vi "read_timer_holding_time.vi"(8 "error in (no error)":errorcluster, 11 "config_file_name":string) -> (0 "error out":errorcluster, 2 "values":cluster{"holding time":dbl}, 3 "config_file_name_out":string)   [LabVIEW 2015]
uses:
  <vilib>/Utility/config.llb/Read Key (String).vi
  <vilib>/Utility/config.llb/NI_LVConfig.lvlib
panel:
  # "Devuelve datos de la sección TIMER del archivo de configuración"
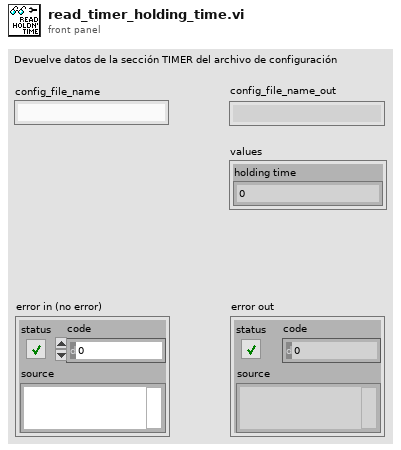
[diagram p1: front panel]
types:
  T1 = typedef "NI_LVConfig.lvlib/Config Data RefNum.ctl" = refnum<k1>
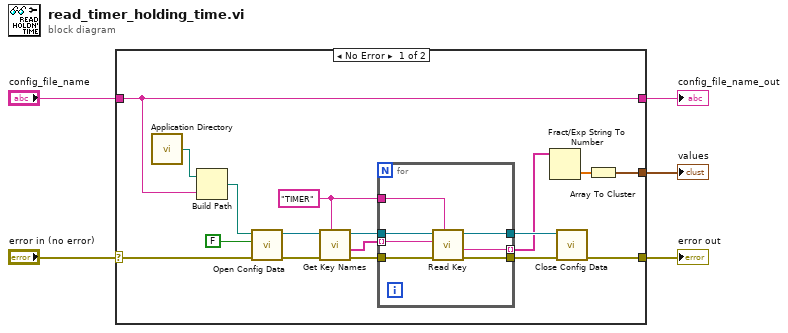
[diagram p0: block diagram]
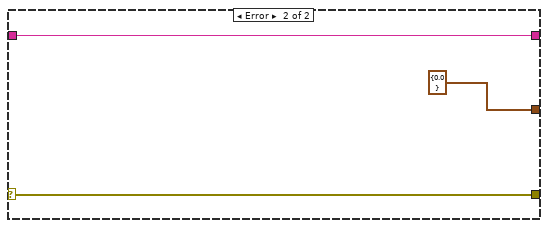
[diagram p2: hidden frame]
diagram:
  n1 = case shown="No Error" "error in (no error)" {
    selector: "error in (no error)" -> [w13 w32]
    tunnel: [w12 w32] -> w5
    tunnel: [w11 w31] -> w3
    tunnel: "config_file_name" -> [w11 w31]
    tunnel: [w6 cluster{"[0]":dbl} {"[0]"=0.0}] -> w1
    frame No Error {
      w18 = "TIMER" ("section")
      n2 = call <vilib>:"Application Directory.vi"() -> ("Application Directory"=w20:path)
      n3 = Build Path(base path=w20, name or relative path=w11) -> (appended path=w19:path)
      n4 = call <vilib>:"Open Config Data.vi"("error in (no error)"=w13, "create file if necessary (T)"=FALSE, "configuration file path"=w19) -> ("error out"=w22:errorcluster, "refnum"=w21:T1)  [unwired: 6 in, 1 out]
      n5 = call <vilib>:"Get Key Names.vi"("section"=w18, "error in (no error)"=w22, "refnum"=w21) -> ("error out"=w16:errorcluster, "key names"=w10:string[], "refnum out"=w17:T1)  [unwired: 5 in, 1 out]
      n6 = for {
        tunnel: w10 -> [w29] mode=indexing
        tunnel: [w28] -> w8 mode=indexing
        tunnel: w18 -> [w27]
        tunnel: w17 -> [w26]
        tunnel: w16 -> [w25]
        tunnel: [w24] -> w15
        tunnel: [w23] -> w14
        n7 = call-poly <vilib>:"Read Key.vi"("section"=w27, "error in (no error)"=w25, "key"=w29, "refnum"=w26) -> ("error out"=w23:errorcluster, "value"=w28:string, "refnum out"=w24:T1)  [unwired: 4 in, 1 out]
      }
      n8 = Fract/Exp String To Number(string=w8) -> (number=w7:dbl[])  [unwired: 3 in, 1 out]
      n9 = call <vilib>:"Close Config Data.vi"("error in (no error)"=w14, "refnum"=w15) -> ("error out"=w12:errorcluster)  [unwired: 8 in, 1 out]
      n10 = Array To Cluster(array=w7) -> (cluster=w6:cluster{"[0]":dbl})
    }
    frame Error {
    }
  }
  "error out" <- w5
  "config_file_name_out" <- w3
  "values" <- w1
